vi "电压输出与采集.vi"() -> ()   [LabVIEW 2014]
uses:
  <vilib>/DAQmx/create/channels.llb/DAQmx Create Channel (AO-Voltage-Basic).vi
  <vilib>/DAQmx/write.llb/DAQmx Write (Analog DBL 1Chan 1Samp).vi
  <vilib>/DAQmx/create/channels.llb/DAQmx Create Channel (AI-Voltage-Basic).vi
  <vilib>/DAQmx/read.llb/DAQmx Read (Analog DBL 1Chan 1Samp).vi
panel:
  in  "physical channels":tag caption="物理通道"
  out "测量电压":dbl
  in  "停止测量":bool
  in  "停止输出":bool
  in  "输出电压":dbl format="%0.2f"
  in  "输出通道":tag
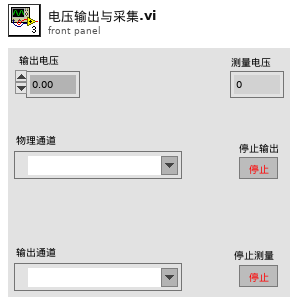
[diagram p1: front panel]
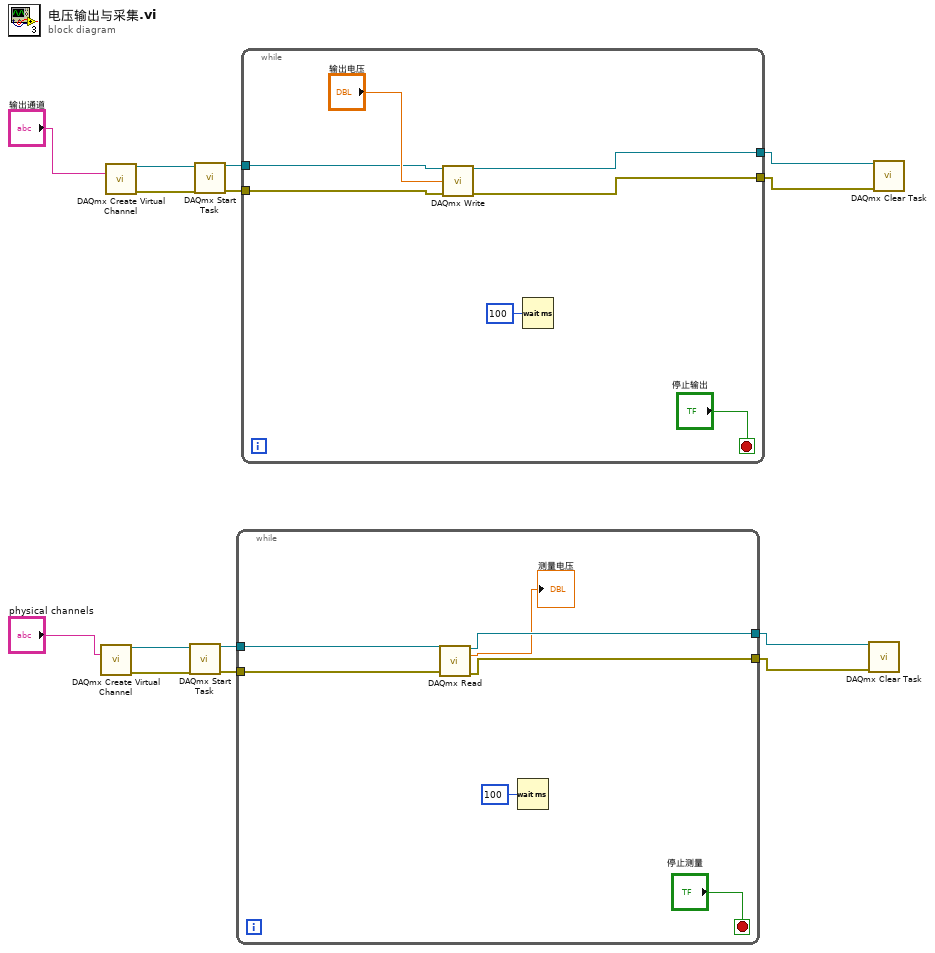
[diagram p0: block diagram]
diagram:
  n1 = call-poly <vilib>:"DAQmx Create Virtual Channel.vi"("physical channels"="physical channels") -> ("task out"=w8:refnum<k21>, "error out"=w7:errorcluster)  [unwired: 13 in]
  n2 = call-poly <vilib>:"DAQmx Create Virtual Channel.vi"("physical channels"="输出通道") -> ("task out"=w14:refnum<k21>, "error out"=w13:errorcluster)  [unwired: 13 in]
  n3 = call <vilib>:"DAQmx Start Task.vi"("task/channels in"=w8, "error in"=w7) -> ("task out"=w6:refnum<k21>, "error out"=w5:errorcluster)  [unwired: 12 in]
  n4 = call <vilib>:"DAQmx Start Task.vi"("task/channels in"=w14, "error in"=w13) -> ("task out"=w12:refnum<k21>, "error out"=w11:errorcluster)  [unwired: 12 in]
  n5 = while {
    tunnel: w6 -> [w19]
    tunnel: w5 -> [w18]
    tunnel: [w17] -> w4
    tunnel: [w16] -> w3
    stop <- "停止测量" stop-if-true
    n6 = call-poly <vilib>:"DAQmx Read.vi"("task/channels in"=w19, "error in"=w18) -> ("task out"=w17:refnum<k21>, "data"=→"测量电压":dbl, "error out"=w16:errorcluster)  [unwired: 11 in]
    n7 = Wait (ms)(milliseconds to wait=u32 100 ("等待时间（毫秒）")) -> ()  [unwired: 1 out]
  }
  n8 = while {
    tunnel: w12 -> [w25]
    tunnel: w11 -> [w24]
    tunnel: [w23] -> w10
    tunnel: [w22] -> w9
    stop <- "停止输出" stop-if-true
    n9 = call-poly <vilib>:"DAQmx Write.vi"("task/channels in"=w25, "data"="输出电压", "error in"=w24) -> ("task out"=w23:refnum<k21>, "error out"=w22:errorcluster)  [unwired: 10 in, 1 out]
    n10 = Wait (ms)(milliseconds to wait=u32 100 ("等待时间（毫秒）")) -> ()  [unwired: 1 out]
  }
  n11 = call <vilib>:"DAQmx Clear Task.vi"("task in"=w4, "error in"=w3) -> ()  [unwired: 13 in, 1 out]
  n12 = call <vilib>:"DAQmx Clear Task.vi"("task in"=w10, "error in"=w9) -> ()  [unwired: 13 in, 1 out]
